vi "SetDriveArcade.vi"(10 "Forward":dbl, 11 "Turn":dbl) -> ()   [LabVIEW 2016]
uses:
  Robot Global Data.vi
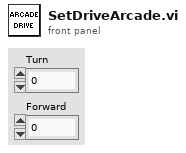
[diagram p1: front panel]
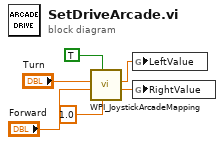
[diagram p0: block diagram]
diagram:
  n1 = call <vilib>:"WPI_JoystickArcadeMapping.vi"("Max Output"=1.0, "Square Inputs"=TRUE, "Y axis value"="Forward", "X axis value"="Turn") -> ("Right Motor Value"=w1:dbl, "Left Motor Value"=w2:dbl)  [unwired: 6 in]
  n2 = global write "Robot Global Data.vi" "LeftValue"(w2) -> ()
  n3 = global write "Robot Global Data.vi" "RightValue"(w1) -> ()
